vi "Do.vi"(8 "error in":errorcluster, 10 "SetTemp Message":refnum<class "SetTemp Message.lvclass">, 11 "Execute":refnum<class "Execute.lvclass">) -> (0 "error out":errorcluster, 2 "SetTemp Message":refnum<class "SetTemp Message.lvclass">, 3 "Execute":refnum<class "Execute.lvclass">)   [LabVIEW 2018, in "QMH_Class.lvlib" / "TestManager.lvlib" / "SetTemp Message.lvclass"]
uses:
  SetTemp Message.lvclass
  Execute_class/Execute.lvclass
  SetTemp Message.lvclass/SetTemp Message.ctl
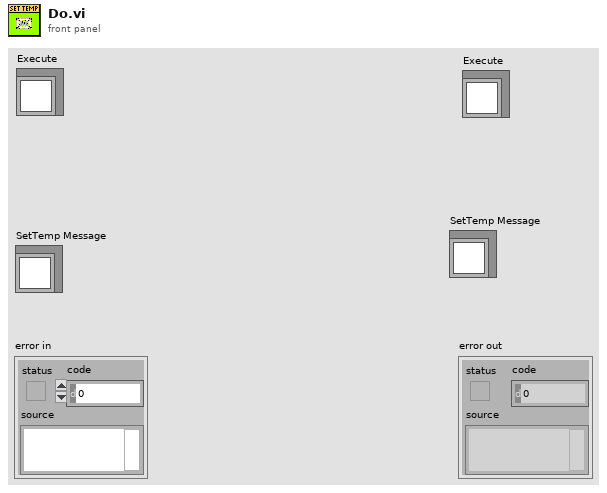
[diagram p1: front panel]
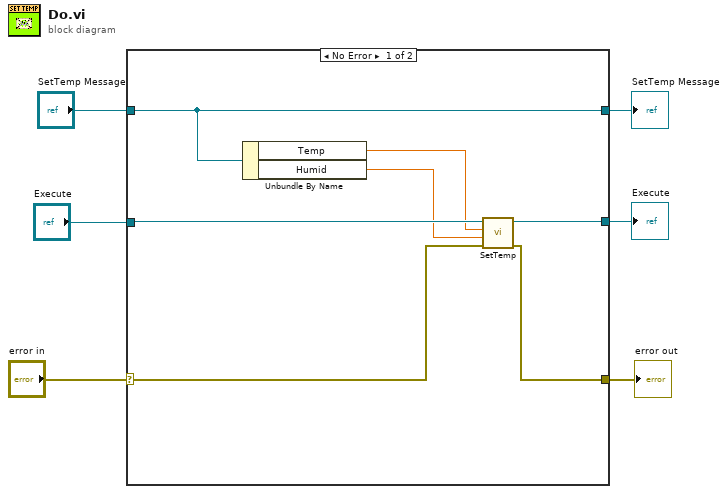
[diagram p0: block diagram]
diagram:
  n1 = case shown="No Error" "error in" {
    selector: "error in" -> [w11 w14]
    tunnel: [w10 w14] -> w5
    tunnel: [w12 w16] -> w4
    tunnel: "Execute" -> [w13 w16]
    tunnel: "SetTemp Message" -> [w9 w15]
    tunnel: [w9 w15] -> w1
    frame No Error {
      n2 = Unbundle By Name(w9) -> ("Temp"=w8:dbl, "Humid"=w7:dbl)
      n3 = call-dynamic "SetTemp.vi"("error in (no error)"=w11, "Humid"=w7, "Temp"=w8, "Execute"=w13) -> ("error out"=w10:errorcluster, "Execute"=w12:refnum<class "Execute.lvclass">)  [unwired: 6 in]
    }
    frame Error {
    }
  }
  "error out" <- w5
  "SetTemp Message" <- w1
  "Execute" <- w4
